vi "001_miernikl_MG.vi"() -> ()   [LabVIEW 2021]
panel:
  out "Poprawana reakcja?":string="Tak"
  out "Czas reakcji [s]":dbl
  out "Prawa dioda":bool=TRUE
  out "Lewa dioda":bool
  in  "Start":bool
  in  "Prawa":bool
  in  "Obie":bool
  in  "Lewa":bool
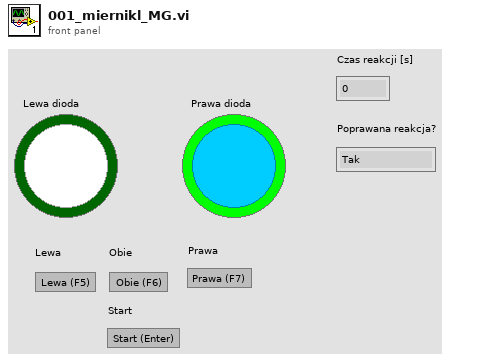
[diagram p1: front panel]
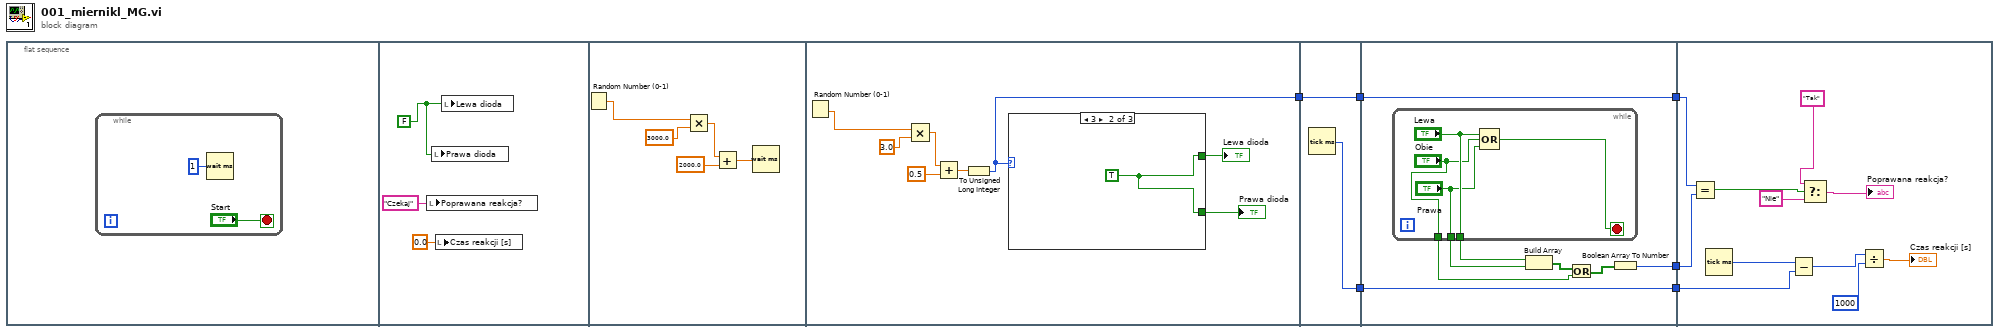
[diagram p0: block diagram]
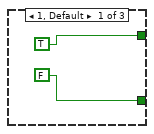
[diagram p2: hidden frame]
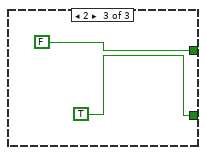
[diagram p3: hidden frame]
diagram:
  n1 = flat-sequence {
    tunnel: [w17] -> w6
    tunnel: w6 -> [w31]
    tunnel: [w31] -> w5
    tunnel: [w30] -> w1
    tunnel: w5 -> [w34]
    tunnel: [w34] -> w4
    tunnel: [w33] -> w3
    tunnel: [w32] -> w2
    tunnel: w1 -> [w32]
    tunnel: w4 -> [w48]
    tunnel: w3 -> [w49]
    tunnel: w2 -> [w47]
    frame #0 {
      n2 = while {
        stop <- "Start" stop-if-true
        n3 = Wait (ms)(milliseconds to wait=u32 1) -> ()  [unwired: 1 out]
      }
    }
    frame #1 {
      w11 = FALSE
      n4 = local write "Poprawana reakcja?"("Czekaj" ("Poprawana reakcja?")) -> ()
      n5 = local write "Prawa dioda"(w11) -> ()
      n6 = local write "Czas reakcji [s]"(0.0 ("Czas reakcji [s]")) -> ()
      n7 = local write "Lewa dioda"(w11) -> ()
    }
    frame #2 {
      n8 = Random Number (0-1)() -> (number: 0 to 1=w16:dbl)
      n9 = Multiply(x=w16, y=3000.0) -> (x*y=w14:dbl)
      n10 = Add(x=w14, y=2000.0) -> (x+y=w12:dbl)
      n11 = Wait (ms)(milliseconds to wait=w12) -> ()  [unwired: 1 out]
    }
    frame #3 {
      n12 = Random Number (0-1)() -> (number: 0 to 1=w24:dbl)
      n13 = Multiply(x=w24, y=3.0) -> (x*y=w22:dbl)
      n14 = Add(x=w22, y=0.5) -> (x+y=w20:dbl)
      n15 = To Unsigned Long Integer(number=w20) -> (unsigned 32bit integer=w17:u32)
      n16 = case shown="3" w17 {
        tunnel: [TRUE w27 FALSE] -> w19
        tunnel: [FALSE w27 TRUE] -> w18
        frame 1, Default {
        }
        frame 3 {
          w27 = TRUE
        }
        frame 2 {
        }
      }
      "Prawa dioda" <- w18
      "Lewa dioda" <- w19
    }
    frame #4 {
      n17 = Tick Count (ms)() -> (millisecond timer value=w30:u32)
    }
    frame #5 {
      n18 = while {
        tunnel: ["Lewa"] -> w39
        tunnel: ["Prawa"] -> w38
        tunnel: ["Obie"] -> w35
        stop <- w43 stop-if-true
        n19 = Compound Arithmetic op=OR("Lewa", "Obie", "Prawa") -> (w43:bool)
      }
      n20 = Build Array(w39, w38) -> (w36:bool[])
      n21 = Or(x=w36, y=w35) -> (x .or. y?=w37:bool[])
      n22 = Boolean Array To Number(Boolean array=w37) -> (number=w33:u32)
    }
    frame #6 {
      n23 = Equal?(x=w48, y=w49) -> (x = y?=w54:bool)
      n24 = Tick Count (ms)() -> (millisecond timer value=w50:u32)
      n25 = Subtract(x=w50, y=w47) -> (x-y=w46:u32)
      n26 = Select(t="Tak", s=w54, f="Nie") -> (s? t:f=→"Poprawana reakcja?":string)
      n27 = Divide(x=w46, y=u32 1000) -> (x/y=→"Czas reakcji [s]":dbl)
    }
  }
